vi "Save File Create Summary Path.vi"(8 "Error In":errorcluster, 9 "Summary":string="_Summary.csv", 10 "Debug":string="_Debug Log.csv", 11 "Debug File Path":path) -> (0 "Error Out":errorcluster, 3 "Path":path)   [LabVIEW 2016, in "Save File.lvlib"]
uses:
  Save File.lvlib
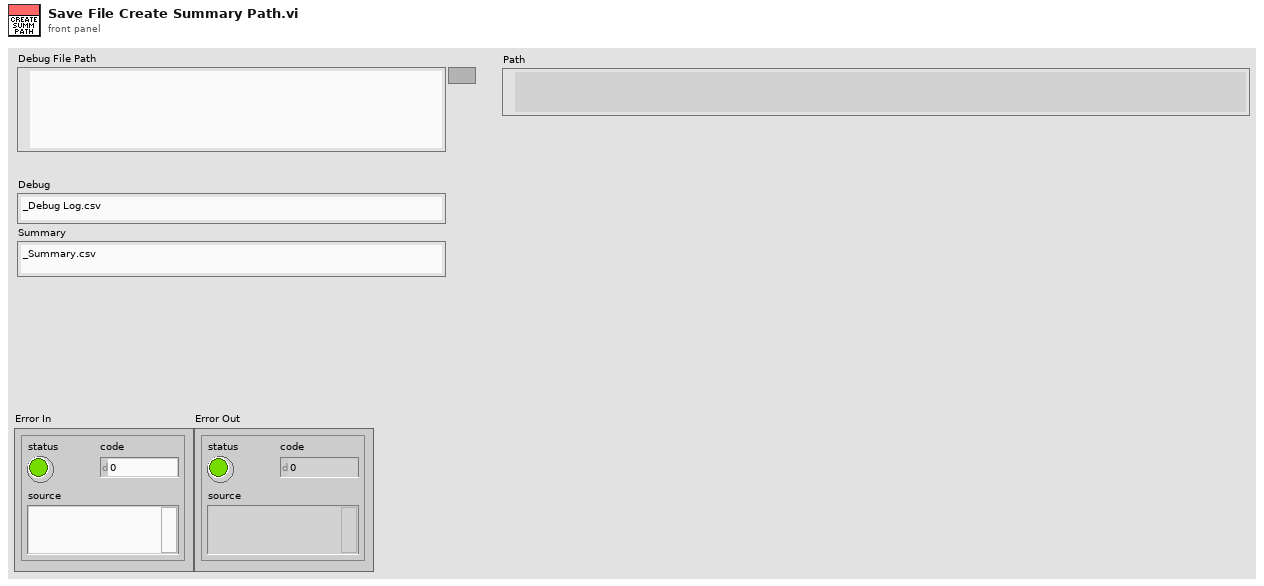
[diagram p1: front panel]
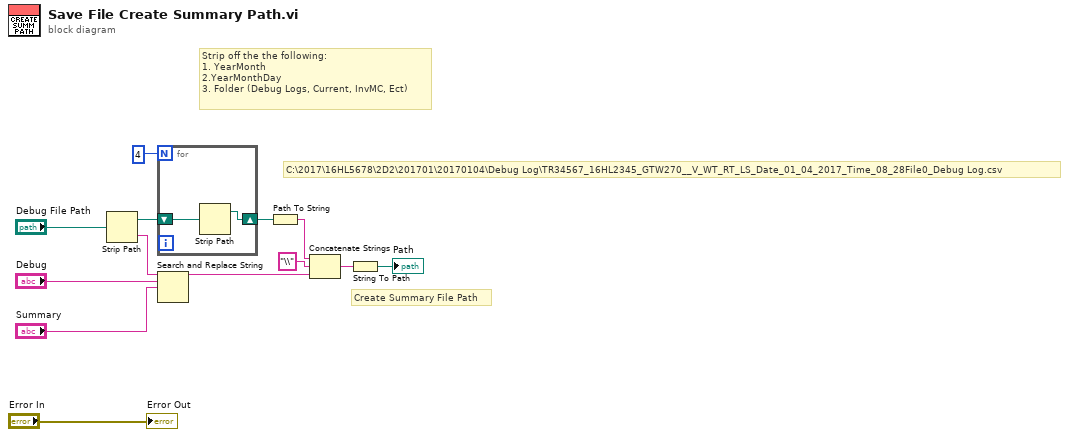
[diagram p0: block diagram]
diagram:
  # "C:\\2017\\16HL5678\\2D2\\201701\\20170104\\Debug Log\\TR34567_16HL2345_GTW270__V_WT_RT_LS_Date_01_04_2017_Time_08_28File0_Debug Log.csv"
  # "Strip off the the following:\n1. YearMonth \n2.YearMonthDay\n3. Folder (Debug Logs, Current, InvMC, Ect)"
  # "Create Summary File Path"
  n1 = Strip Path(path="Debug File Path") -> (stripped path=w11:path, name=w5:string)
  n2 = for {
    N: 4 -> [_]
    shift-right: [w14] -> w12
    shift-left: w11 -> [w15]
    n3 = Strip Path(path=w15) -> (stripped path=w14:path)  [unwired: 1 out]
  }
  n4 = Search and Replace String(input string=w5, search string="Debug", replace string="Summary") -> (result string=w9:string)  [unwired: 5 in, 3 out]
  n5 = Path To String(path=w12) -> (string=w7:string)
  n6 = Concatenate Strings(w7, "\\" ("string"), w9) -> (w10:string)
  n7 = String To Path(string=w10) -> (path=→"Path":path)
  "Error Out" <- "Error In"
